vi "ContractRelaxTimer.vi"() -> ()   [LabVIEW 2014]
panel:
  in  "Relax Duration (ms)":u32
  in  "Contraction Duration (ms)":u32
  out "Relax":bool
  out "Contract":bool
  out "Rep Number":i32
  out "Set Number":i32
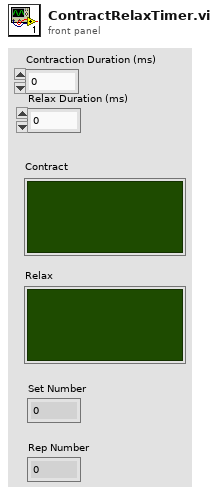
[diagram p1: front panel]
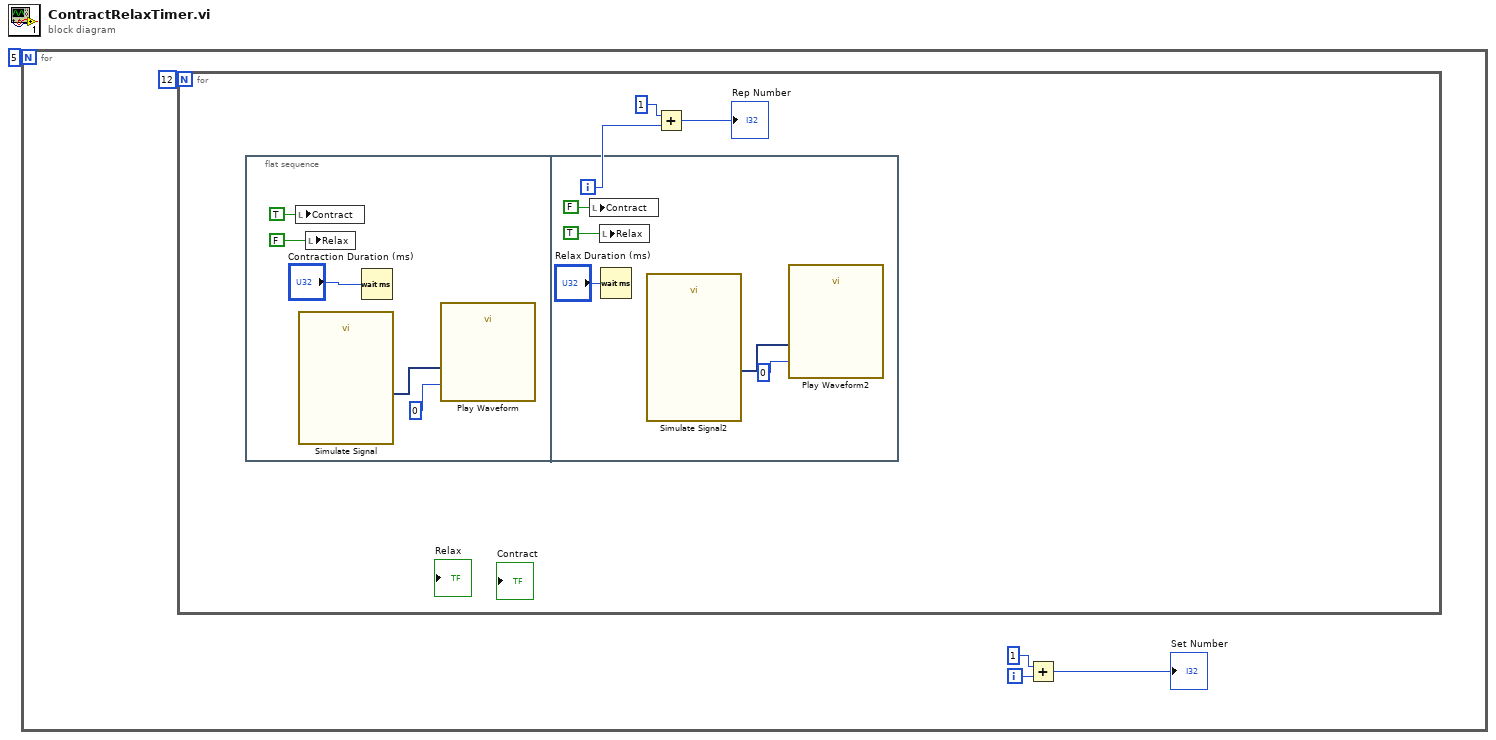
[diagram p0: block diagram]
diagram:
  n1 = for {
    N: 5 -> [_]
    i -> [w3]
    n2 = for {
      N: 12 -> [_]
      i -> [w6]
      n3 = flat-sequence {
        frame #0 {
          n4 = local write "Contract"(TRUE ("Boolean")) -> ()
          n5 = call "Simulate Signal"() -> ("Sine"=w12:dynamicdata)  [unwired: 14 in, 1 out]
          n6 = local write "Relax"(FALSE ("Boolean")) -> ()
          n7 = Wait (ms)(milliseconds to wait="Contraction Duration (ms)") -> ()  [unwired: 1 out]
          n8 = call "Play Waveform"("Device"=u32 0, "Data"=w12) -> ()  [unwired: 17 in, 1 out]
        }
        frame #1 {
          n9 = local write "Contract"(FALSE ("Boolean")) -> ()
          n10 = local write "Relax"(TRUE ("Boolean")) -> ()
          n11 = Wait (ms)(milliseconds to wait="Relax Duration (ms)") -> ()  [unwired: 1 out]
          n12 = call "Simulate Signal2"() -> ("Sine"=w18:dynamicdata)  [unwired: 14 in, 1 out]
          n13 = call "Play Waveform2"("Device"=u32 0, "Data"=w18) -> ()  [unwired: 17 in, 1 out]
        }
      }
      n14 = Add(x=1, y=w6) -> (x+y=→"Rep Number":i32)
    }
    n15 = Add(x=1, y=w3) -> (x+y=→"Set Number":i32)
  }
